vi "SUB_WR_COM1_CbyCFindString_timeout.vi"(4 "Begin time":dbl, 5 "Find this String":string, 6 "Timeout Seccond":dbl, 7 "cmd string":string, 8 "duplicate VISA resource name 2":refnum<visa-resource-name>) -> (0 "VISA out":refnum<visa-resource-name>, 1 "Output String":string, 2 "spent seconds":dbl, 3 "Found String":bool)   [LabVIEW 2011]
panel:
  out "String":string
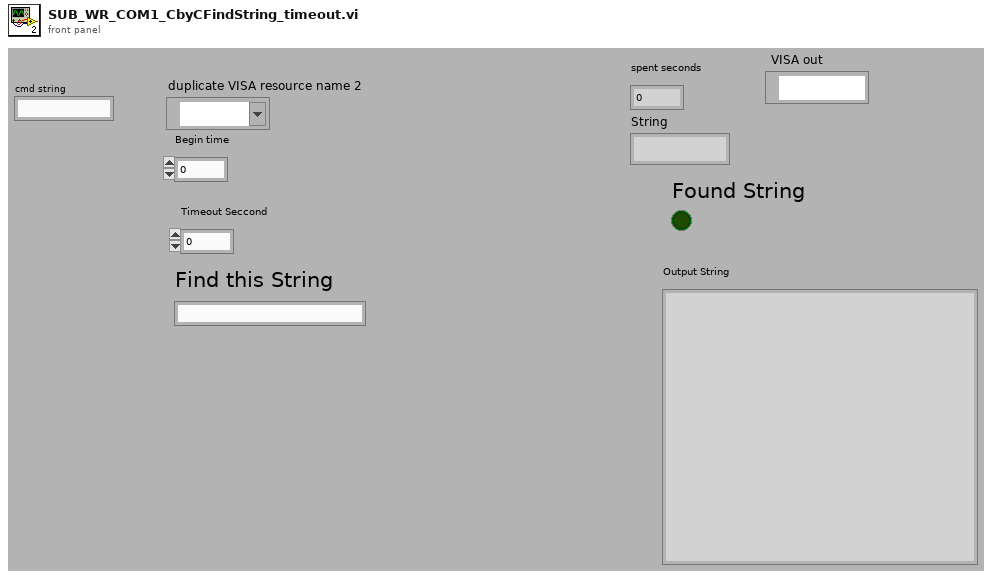
[diagram p1: front panel]
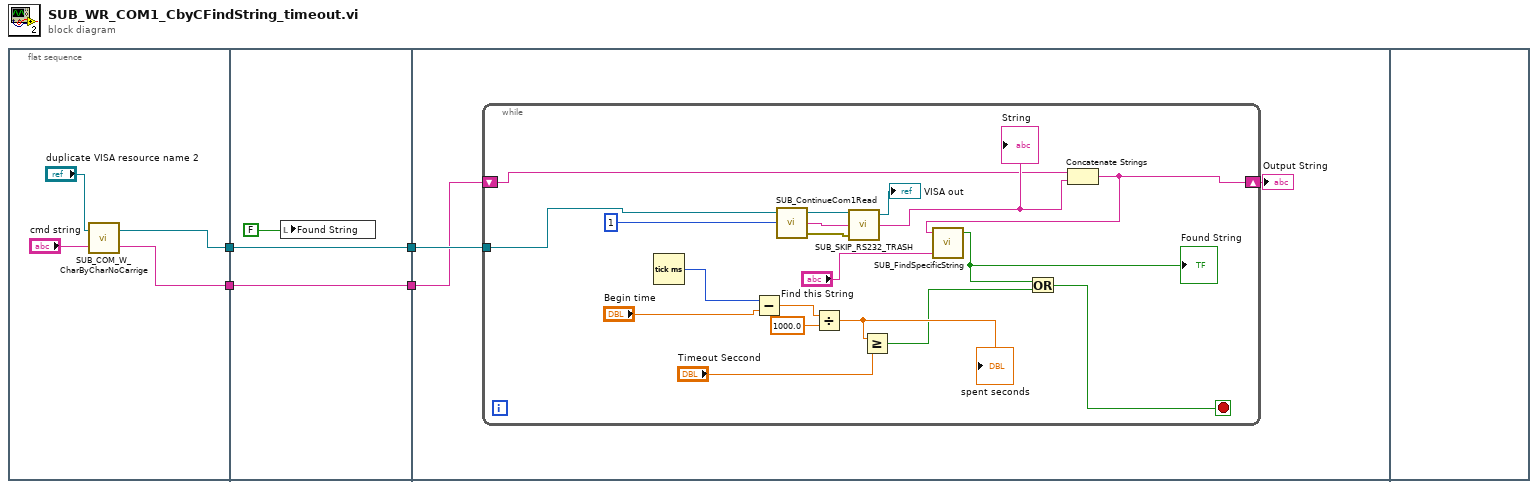
[diagram p0: block diagram]
diagram:
  n1 = flat-sequence {
    tunnel: [w7] -> w3
    tunnel: [w5] -> w1
    tunnel: [w10] -> w4
    tunnel: w3 -> [w10]
    tunnel: [w9] -> w2
    tunnel: w1 -> [w9]
    tunnel: w4 -> [w13]
    tunnel: w2 -> [w12]
    frame #0 {
      n2 = call "SUB_COM_W_CharByCharNoCarrige.vi"("cmd string"="cmd string", "duplicate VISA resource name"="duplicate VISA resource name 2") -> ("OUT string"=w5:string, "VISA resource OUT"=w7:refnum<visa-resource-name>)
    }
    frame #1 {
      n3 = local write "Found String"(FALSE) -> ()
    }
    frame #2 {
      n4 = while {
        shift-right: [w15] -> w14
        shift-left: w12 -> [w20]
        tunnel: w13 -> [w17]
        stop <- w23 stop-if-true
        n5 = Tick Count (ms)() -> (millisecond timer value=w19:u32)
        n6 = Subtract(x=w19, y="Begin time") -> (x-y=w29:dbl)
        n7 = call "SUB_ContinueCom1Read.vi"("Numeric"=1, "duplicate VISA resource name 2"=w17) -> ("error out"=w31:errorcluster, "String"=w32:string, "duplicate VISA resource name"=w33:refnum<visa-resource-name>)  [unwired: 1 in]
        n8 = Divide(x=w29, y=1000.0) -> (x/y=w27:dbl)
        "spent seconds" <- w27
        n9 = call "SUB_SKIP_RS232_TRASH.vi"("error out 2"=w31, "read buffer"=w32, "duplicate VISA resource name 2"=w33) -> ("String"=w21:string, "duplicate VISA resource name"=→"VISA out":refnum<visa-resource-name>)  [unwired: 1 out]
        "String" <- w21
        n10 = Greater Or Equal?(x=w27, y="Timeout Seccond") -> (x >= y?=w24:bool)
        n11 = Concatenate Strings(w20, w21) -> (w15:string)
        n12 = call "SUB_FindSpecificString.vi"("Find this String"="Find this String", "String data"=w15) -> ("Found"=w25:bool)  [unwired: 2 in, 1 out]
        "Found String" <- w25
        n13 = Or(x=w25, y=w24) -> (x .or. y?=w23:bool)
      }
      "Output String" <- w14
    }
    frame #3 {
    }
  }
